vi "GenerateTests.vi"() -> ()   [LabVIEW 2014]
uses:
  GUI_StateDataTD.ctl
  Classes/TestCase/TestCase.lvclass/TestCase.ctl
  <vilib>/NI/AMC/Read Termination Message.vi
  <vilib>/NI/AMC/Create Single Message.vi
  <vilib>/NI/AMC/Update Message Routing Info.vi
  <vilib>/NI/AMC/Send Message.vi
  <vilib>/NI/AMC/Globals.vi
  <vilib>/NI/AMC/AMC.lvlib
  Classes/TestCase/TestCase.lvclass
  <resource>/objmgr/DOMUserDefRef.rc
panel:
  in  "VI":path
  in  "Run VI":bool
  in  "stop":bool
  out "XML":string
  in  "name":string
  in  "state variables":T1
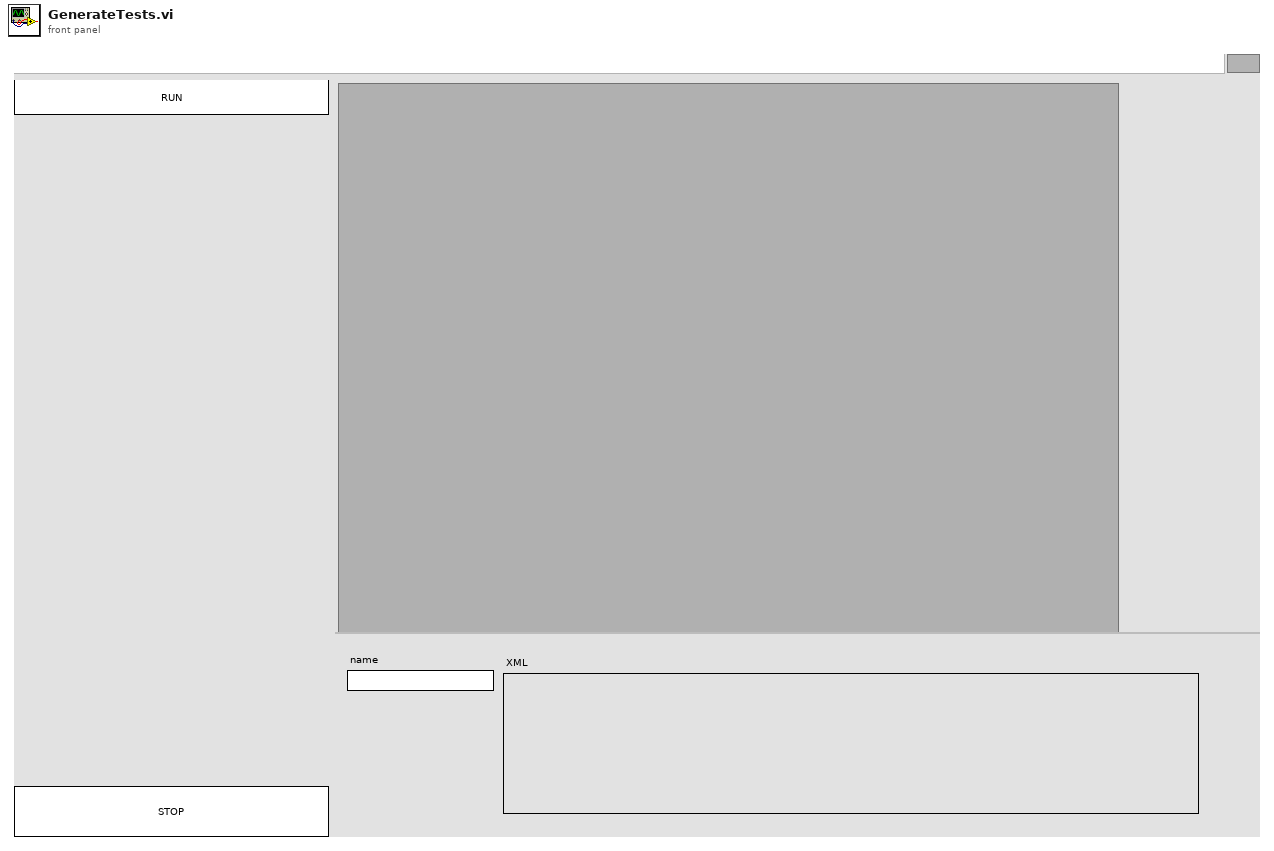
[diagram p1: front panel]
types:
  T1 = typedef "GUI_StateDataTD.ctl" = cluster{"CurrentFile":path, "VI Refnum":refnum<vi>}
  T2 = typedef "AMC.lvlib/Message Queue.ctl" = refnum<queue>
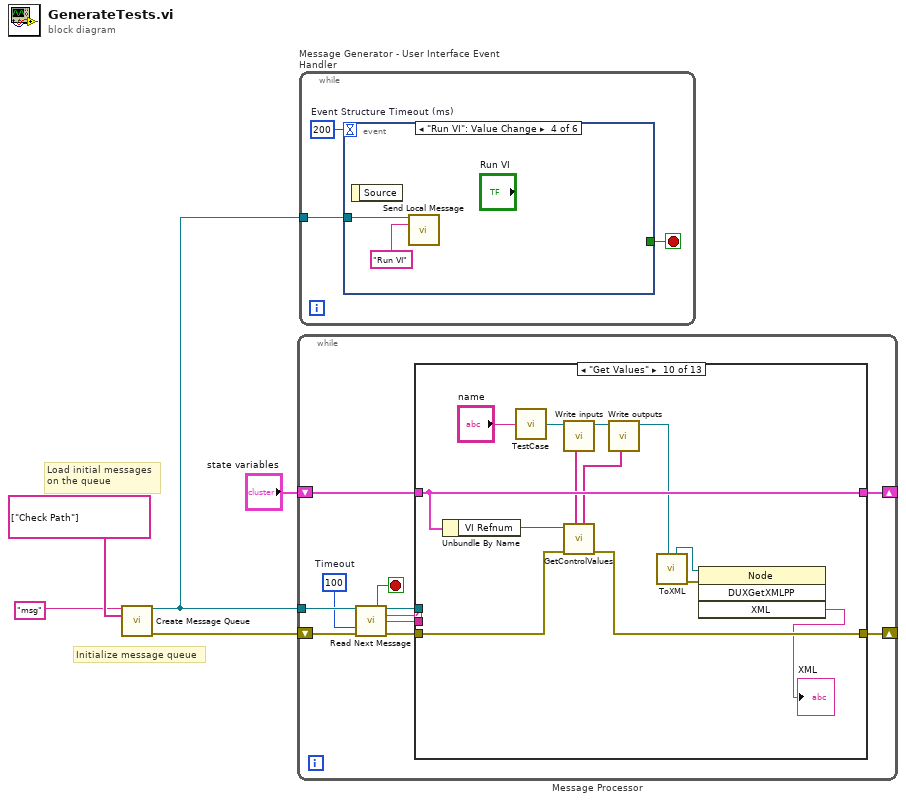
[diagram p0: block diagram]
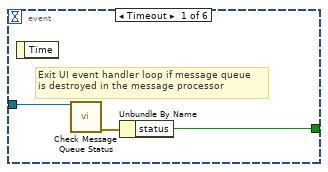
[diagram p2: hidden frame]
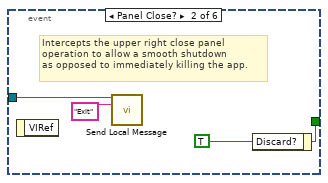
[diagram p3: hidden frame]
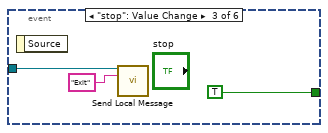
[diagram p4: hidden frame]
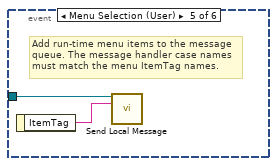
[diagram p5: hidden frame]
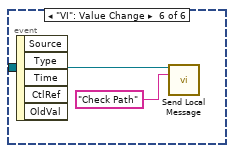
[diagram p6: hidden frame]
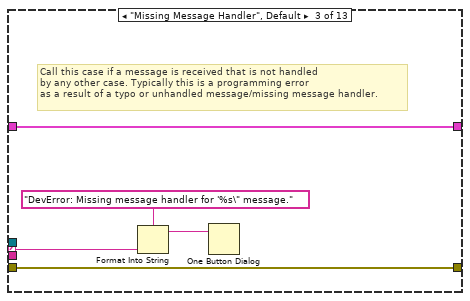
[diagram p9: hidden frame]
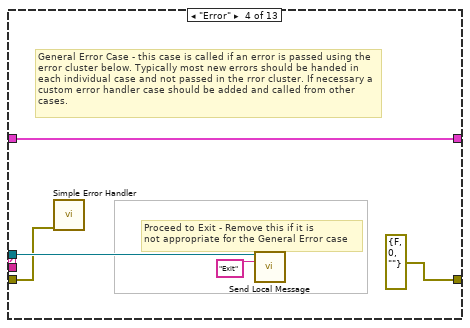
[diagram p10: hidden frame]
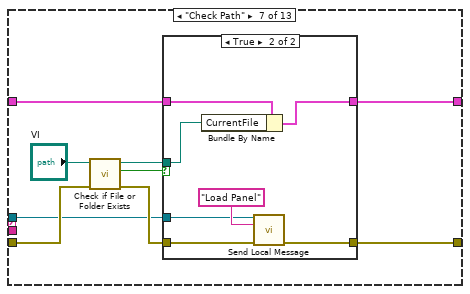
[diagram p13: hidden frame]
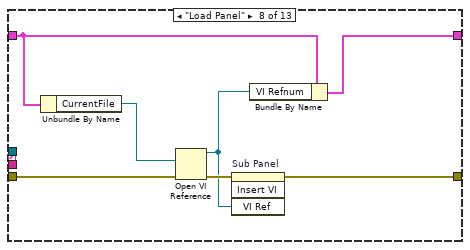
[diagram p15: hidden frame]
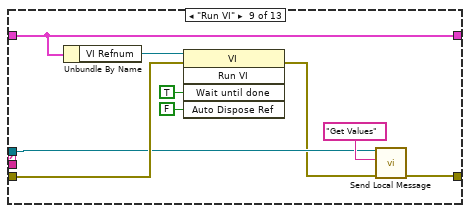
[diagram p16: hidden frame]
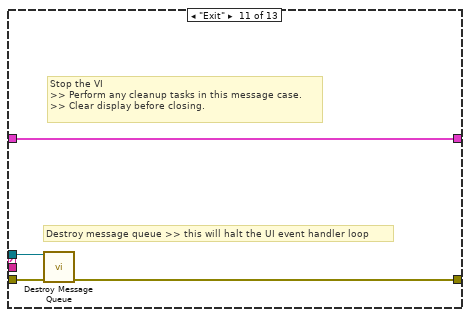
[diagram p17: hidden frame]
diagram:
  # "Initialize message queue"
  # "Load initial messages\non the queue"
  n1 = call <vilib>:"Create Message Queue.vi"("message queue name"="msg", "initial message names"=string[] ["Check Path"]) -> ("message queue out"=w4:T2, "error out"=w3:errorcluster)  [unwired: 12 in]
  n2 = while "Message Processor" {
    shift-left: w3 -> [w10]
    shift-right: [w14] -> _
    tunnel: w4 -> [w11]
    shift-left: "state variables" -> [w16]
    shift-right: [w15] -> _
    stop <- w13 stop-if-true
    w6 = 100  # Timeout
    n3 = call <vilib>:"Read Next Message.vi"("message queue in"=w11, "timeout (1 ms)"=w6, "error in"=w10) -> ("exit process?"=w13:bool, "message queue out"=w12:T2, "message name"=w8:string, "message value"=w7:string, "error out"=w9:errorcluster)  [unwired: 5 in, 3 out]
    n4 = case shown="\"Get Values\"" w8 {
      selector: w8 -> [_ _ w23 _ _ _ _ _ _ _ _ _ _]
      tunnel: [w18 w20 w25 w30 w32 w34 w36 w53 w68 w81 w85 w87 w88] -> w15
      tunnel: w16 -> [w18 w20 w25 w30 w32 w34 w37 w55 w68 w81 w85 w87 w88]
      tunnel: w12 -> [_ _ _ w28 _ _ w35 _ w62 _ w83 _ _]
      tunnel: w9 -> [w17 w19 w24 w26 w31 w33 w43 w59 w66 w80 w84 w86 w89]
      tunnel: [w17 w19 w24 errorcluster {"status"=FALSE, "code"=0, "source"=""} ("error out") w31 w33 w39 w56 w61 w79 w82 w86 w89] -> w14
      tunnel: w7 -> [_ _ _ _ _ _ _ _ _ _ _ _ _]
      frame "---------- Framework Operations ----------" {
        # "Dummy case to add a seperator in the Case Structure menu"
      }
      frame "", "Idle" {
      }
      frame "Missing Message Handler", Default {
        # "Call this case if a message is received that is not handled \nby any other case. Typically this is a programming error\nas a result of a typo or unhandled message/missing message handler."
        n5 = Format Into String(format string="DevError: Missing message handler for '%s\" message." ("message"), w23) -> (resulting string=w21:string)  [unwired: 2 in, 1 out]
        n6 = One Button Dialog(message=w21) -> ()  [unwired: 2 out]
      }
      frame "Error" {
        # "Proceed to Exit - Remove this if it is\nnot appropriate for the General Error case"
        # "General Error Case - this case is called if an error is passed using the error cluster below. Typically most new errors should be handed in each individual case and not passed in the rror cluster. If necessary a custom error handler case should be added and called from other cases."
        n7 = call <vilib>:"Simple Error Handler.vi"("error in (no error)"=w26) -> ()  [unwired: 1 in, 8 out]
        n8 = call <vilib>:"Send Local Message.vi"("message queue in"=w28, "message name"="Exit") -> ()  [unwired: 11 in, 3 out]
      }
      frame "---------- Generic Operations ----------" {
        # "Dummy case to add a seperator in the Case Structure menu"
      }
      frame "Initialize" {
      }
      frame "Check Path" {
        n9 = call <vilib>:"Check if File or Folder Exists.vi"("error in (no error)"=w43, "path"="VI") -> ("error out"=w40:errorcluster, "file or folder exists?"=w41:bool, "dup path"=w38:path)  [unwired: 7 in]
        n10 = case shown="True" w41 {
          tunnel: w40 -> [w45 w51]
          tunnel: [w45 w50] -> w39
          tunnel: w38 -> [_ w48]
          tunnel: w37 -> [w44 w49]
          tunnel: [w44 w47] -> w36
          tunnel: w35 -> [_ w46]
          frame False {
          }
          frame True {
            n11 = Bundle By Name(cluster=w49, "CurrentFile"=w48) -> (w47:T1)
            n12 = call <vilib>:"Send Local Message.vi"("message queue in"=w46, "message name"="Load Panel", "error in"=w51) -> ("error out"=w50:errorcluster)  [unwired: 10 in, 2 out]
          }
        }
      }
      frame "Load Panel" {
        n13 = Unbundle By Name(w55) -> ("CurrentFile"=w58:path)
        n14 = Open VI Reference(vi path=w58, error in (no error)=w59) -> (vi reference=w54:refnum<vi>, error out=w57:errorcluster)  [unwired: 4 in]
        n15 = invoke on="Sub Panel" class="SubPanel" method="Insert VI"(error in=w57, "VI Ref"=w54) -> (error out=w56:errorcluster)  [unwired: 2 in, 3 out]
        n16 = Bundle By Name(cluster=w55, "VI Refnum"=w54) -> (w53:T1)
      }
      frame "Run VI" {
        n17 = Unbundle By Name(w68) -> ("VI Refnum"=w67:refnum<vi>)
        n18 = invoke class="VI" method="Run VI"(reference=w67, error in=w66, "Wait until done"=TRUE ("Wait Until Done"), "Auto Dispose Ref"=FALSE ("Auto Dispose Reference")) -> (error out=w60:errorcluster)  [unwired: 1 in, 4 out]
        n19 = call <vilib>:"Send Local Message.vi"("message queue in"=w62, "message name"="Get Values", "error in"=w60) -> ("error out"=w61:errorcluster)  [unwired: 10 in, 2 out]
      }
      frame "Get Values" {
        n20 = Unbundle By Name(w81) -> ("VI Refnum"=w78:refnum<vi>)
        n21 = call "TestCase.vi"("name"="name") -> ("TestCase out"=w76:refnum<class "TestCase.lvclass">)
        n22 = call "GetControlValues.vi"("error in"=w80, "VI Refnum"=w78) -> ("error out"=w79:errorcluster, "outputs"=w73:string[], "inputs"=w75:string[])  [unwired: 5 in]
        n23 = call "Write inputs.vi"("inputs"=w75, "TestCase in"=w76) -> ("TestCase out"=w74:refnum<class "TestCase.lvclass">)  [unwired: 7 in]
        n24 = call "Write outputs.vi"("outputs"=w73, "TestCase in"=w74) -> ("TestCase out"=w72:refnum<class "TestCase.lvclass">)  [unwired: 7 in]
        n25 = call "ToXML.vi"("TestCase"=w72) -> ("error out"=w71:errorcluster, "TestCase element"=w69:refnum<k20>)  [unwired: 6 in, 1 out]
        n26 = invoke class="Node" method="DUXGetXMLPP"(reference=w69, error in=w71) -> ("XML"=→"XML":string)  [unwired: 2 in, 3 out]
      }
      frame "Exit" {
        # "Destroy message queue >> this will halt the UI event handler loop"
        # "Stop the VI\n>> Perform any cleanup tasks in this message case.\n>> Clear display before closing."
        n27 = call <vilib>:"Destroy Message Queue.vi"("message queue in"=w83, "error in"=w84) -> ("error out"=w82:errorcluster)  [unwired: 11 in, 2 out]
      }
      frame "---------- Application Operations ----------" {
        # "Dummy case to add a seperator in the Case Structure menu"
      }
      frame "Process Data" {
      }
    }
  }
  n28 = while "Message Generator - User Interface Event Handler" {
    tunnel: w4 -> [w90]
    stop <- w91 stop-if-true
    w92 = 200  # Event Structure Timeout (ms)
    n29 = event shown="[3] \"Run VI\": Value Change" {
      selector: _ -> [_ _ _ _ _ _]
      dyn-events: _ -> [_ _ _ _ _ _]
      timeout: w92 -> [_ _ _ _ _ _]
      tunnel: [w93 w98 TRUE ("Discard?") _ _ _] -> w91
      tunnel: w90 -> [w94 w96 w99 w102 w104 w107]
      event Timeout {
        # "Exit UI event handler loop if message queue\nis destroyed in the message processor"
        n30 = event-data() -> ()  [unwired: 2 out]
        n31 = call <vilib>:"Check Message Queue Status.vi"("message queue in"=w94) -> ("error out"=w95:errorcluster)  [unwired: 10 in, 4 out]
        n32 = Unbundle By Name(w95) -> ("status"=w93:bool)
      }
      event Panel Close? {
        w98 = TRUE ("Discard?")
        # "Intercepts the upper right close panel\noperation to allow a smooth shutdown\nas opposed to immediately killing the app."
        n33 = event-data() -> ()  [unwired: 2 out]
        n34 = call <vilib>:"Send Local Message.vi"("message queue in"=w96, "message name"="Exit") -> ()  [unwired: 11 in, 3 out]
        n35 = event-data("Discard?"=w98) -> ()  [unwired: 1 in, 1 out]
      }
      event "stop": Value Change {
        n36 = event-data() -> ()  [unwired: 2 out]
        n37 = call <vilib>:"Send Local Message.vi"("message queue in"=w99, "message name"="Exit") -> ()  [unwired: 11 in, 3 out]
      }
      event "Run VI": Value Change {
        n38 = event-data() -> ()  [unwired: 2 out]
        n39 = call <vilib>:"Send Local Message.vi"("message queue in"=w102, "message name"="Run VI") -> ()  [unwired: 11 in, 3 out]
      }
      event Menu Selection (User) {
        # "Add run-time menu items to the message\nqueue. The message handler case names must match the menu ItemTag names."
        n40 = event-data() -> ("ItemTag"=w105:string)  [unwired: 1 out]
        n41 = call <vilib>:"Send Local Message.vi"("message queue in"=w104, "message name"=w105) -> ()  [unwired: 11 in, 3 out]
      }
      event "VI": Value Change {
        n42 = event-data() -> ()  [unwired: 6 out]
        n43 = call <vilib>:"Send Local Message.vi"("message queue in"=w107, "message name"="Check Path") -> ()  [unwired: 11 in, 3 out]
      }
    }
  }
